vi "SubPanel_JSON_PowerConfiguration.vi"(3 "error_input":errorcluster, 4 "ColorPalette":T4=[16711686, 65351, 8978420, 14474240, 16139007, 16752640, 8958719, 16758973, 16777215, 46792, 11992992, 12961221, 16763690, 12600063, 16711835, 2953983, 40796, 13111296, 13352613, 9221011, 12964076, 12819897, 65442, 16776704, 14540253, 16740729, 10658047, 10813344, 16753521, 13413843, 8691115, 10339240, 14401205, 16746704, 7467519, 16775978, 13872558, 11387603, 13354405, 10420227, 13107364, 4060, 35208, 11817216, 7566080, 40796, 7539456, 2837073, 6372186, 7499083, 10648702, 16757152], 5 "VISAPowerInfoInputArray":T3[](array[typedef]), 6 "DCPowerInformationClusterArray_Input":T2[](array[typedef])) -> (0 "error output":errorcluster, 1 "VISAPowerInfoOutputArray":T3[](array[typedef]), 2 "DCPower_byInstrument_output":T1(array[cluster]))   [LabVIEW 2019]
uses:
  Controls/PlotColorArray.ctl
  Controls/VISA_power_Control.ctl
  Controls/DCPowerBlock_byInstrument_Control.ctl
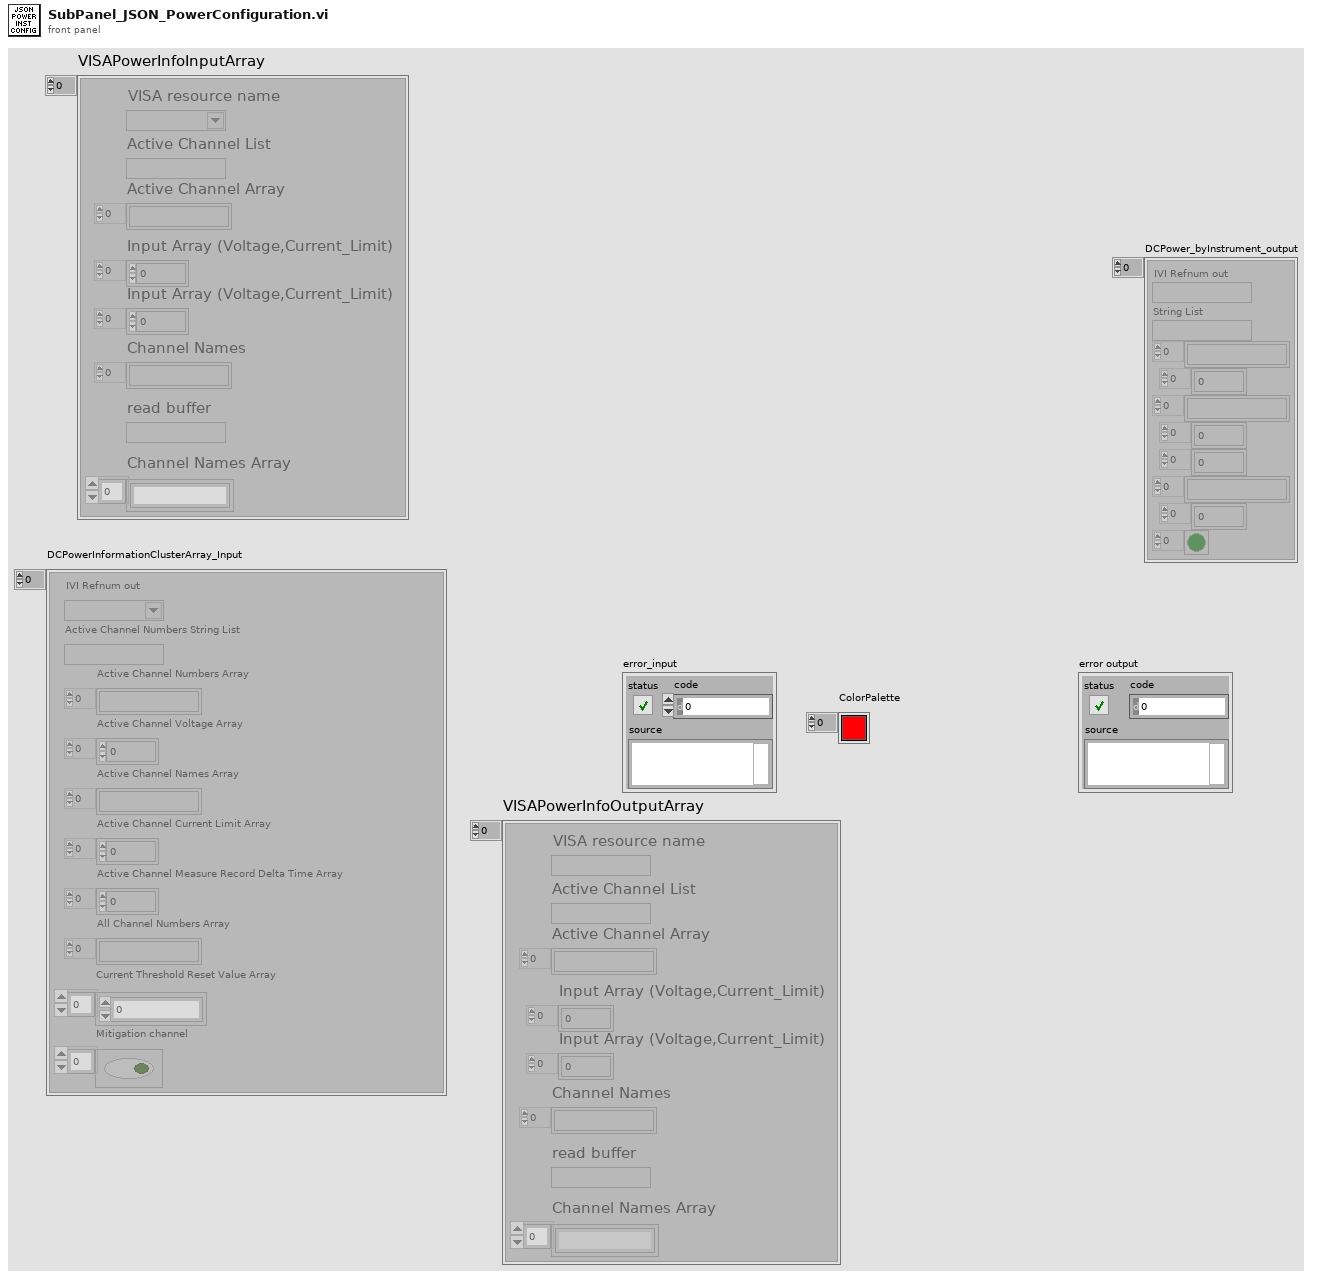
[diagram p1: front panel]
types:
  T1 = cluster{"IVI Refnum out":refnum<k15>, "String List":string, string[], dbl[], string[], dbl[], dbl[], string[], dbl[], bool[]}[]
  T2 = typedef "DCPowerBlock_byInstrument_Control.ctl" = cluster{"IVI Refnum out":refnum<k15>, "Active Channel Numbers String List":string, "Active Channel Numbers Array":string[], "Active Channel Voltage Array":dbl[], "Active Channel Names Array":string[], "Active Channel Current Limit Array":dbl[], "Active Channel Measure Record Delta Time Array":dbl[], "All Channel Numbers Array":string[], "Current Threshold Reset Value Array":dbl[], "Mitigation channel":bool[]}
  T3 = typedef "VISA_power_Control.ctl" = cluster{"VISA resource name":refnum<visa-resource-name>, "Active Channel List":string, "Active Channel Array":string[], "Input Array (Voltage,Current_Limit)":dbl[], "Input Array (Voltage,Current_Limit)":dbl[], "Channel Names":string[], "read buffer":string, "Channel Names Array":string[]}
  T4 = typedef "PlotColorArray.ctl" = u32[]
  T5 = cluster{"IVI Refnum out":refnum<k15>, "Active Channel Numbers String List":string, "Active Channel Numbers Array":string[], "Active Channel Voltage Array":dbl[], "Active Channel Names Array":string[], "Active Channel Current Limit Array":dbl[], "Active Channel Measure Record Delta Time Array":dbl[], "All Channel Numbers Array":string[], "Current Threshold Reset Value Array":dbl[], "Mitigation channel":bool[]}
  T6 = cluster{"IVI Refnum out":refnum<k15>, string, "voltage level channel 23":dbl, "Channel Name 23":string, "Current Limit":dbl, "Measure Record dt":dbl, string, "Current Threshold Reset Value Array":dbl, "Mitigation Channel":bool}[]
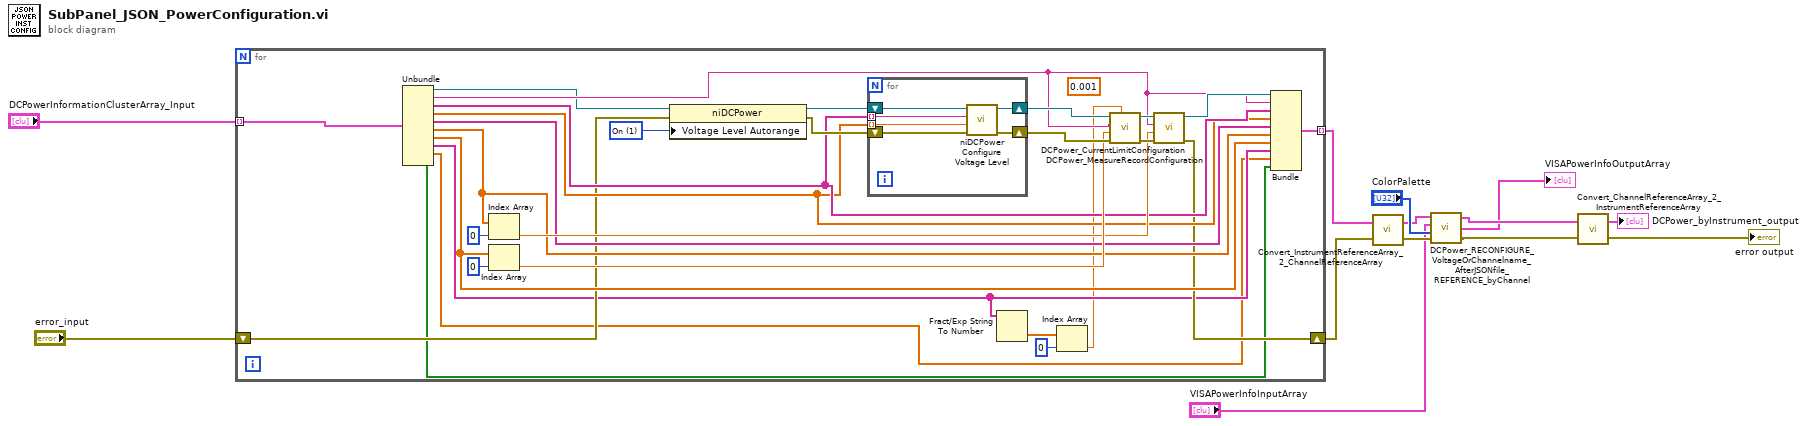
[diagram p0: block diagram]
diagram:
  n1 = for {
    tunnel: "DCPowerInformationClusterArray_Input" -> [w42] mode=indexing
    shift-right: [w20] -> w13
    shift-left: "error_input" -> [w21]
    tunnel: [w23] -> w12 mode=indexing
    (unwired) 0.001 ("Aperture Time")
    w41 = 1 items=["Off", "On"] ("Source:DC Voltage:Voltage Level Autorange")
    n2 = Unbundle(w42) -> ("IVI Refnum out"=w22:refnum<k15>, "Active Channel Numbers String List"=w29:string, "Active Channel Numbers Array"=w28:string[], "Active Channel Voltage Array"=w27:dbl[], "Active Channel Names Array"=w26:string[], "Active Channel Current Limit Array"=w25:dbl[], "Active Channel Measure Record Delta Time Array"=w24:dbl[], "All Channel Numbers Array"=w19:string[], "Current Threshold Reset Value Array"=w15:dbl[], "Mitigation channel"=w14:bool[])
    n3 = Index Array(array=w25, index=0) -> (element=w31:dbl)
    n4 = Index Array(array=w24, index=0) -> (element=w34:dbl)
    n5 = property class="niDCPower"(reference=w22, error in=w21, "Voltage Level Autorange"=w41) -> (reference out=w40:refnum<k15>, error out=w39:errorcluster)
    n6 = for {
      shift-right: [w48] -> w38
      shift-left: w39 -> [w46]
      shift-right: [w45] -> w37
      shift-left: w40 -> [w47]
      tunnel: w28 -> [w44] mode=indexing
      tunnel: w27 -> [w43] mode=indexing
      n7 = call <instrlib>:"niDCPower Configure Voltage Level.vi"("error in (no error)"=w46, "voltage level"=w43, "channel name"=w44, "instrument handle"=w47) -> ("error out"=w48:errorcluster, "instrument handle out"=w45:refnum<k15>)  [unwired: 6 in]
    }
    n8 = Fract/Exp String To Number(string=w19) -> (number=w17:dbl[])  [unwired: 3 in, 1 out]
    n9 = Index Array(array=w17, index=0) -> (element=w16:dbl)
    n10 = call "DCPower_MeasureRecordConfiguration.vi"("Aperture Time"=w16, "error in (no error)"=w38, "Measure Record Length"=w34, "Active Channel Numbers String"=w29, "IVI Refnum in"=w37) -> ("error out"=w33:errorcluster, "IVI Refnum out"=w32:refnum<k15>)  [unwired: 4 in, 1 out]
    n11 = call "DCPower_CurrentLimitConfiguration.vi"("error in (no error)"=w33, "current limit"=w31, "Active Channel Numbers String"=w29, "IVI Refnum in"=w32) -> ("error out"=w20:errorcluster, "IVI Refnum out"=w30:refnum<k15>)  [unwired: 6 in]
    n12 = Bundle("IVI Refnum out"=w30, "Active Channel Numbers String List"=w29, "Active Channel Numbers Array"=w28, "Active Channel Voltage Array"=w27, "Active Channel Names Array"=w26, "Active Channel Current Limit Array"=w25, "Active Channel Measure Record Delta Time Array"=w24, "All Channel Numbers Array"=w19, "Current Threshold Reset Value Array"=w15, "Mitigation channel"=w14) -> (w23:T5)  [unwired: 1 in]
  }
  n13 = call "Convert_InstrumentReferenceArray_2_ChannelReferenceArray.vi"("error in (no error)"=w13, "DCPowerInformationClusterArray_Input"=w12) -> ("error out"=w9:errorcluster, "DCPowerInformationArrayOutput_byChannel"=w2:T6)
  n14 = call "DCPower_RECONFIGURE_VoltageOrChannelname_AfterJSONfile_REFERENCE_byChannel.vi"("error in"=w9, "ColorPalette"="ColorPalette", "VISAPowerInfoInputArray"="VISAPowerInfoInputArray", "DCPowerInformationArrayOutput_byChannel_input"=w2) -> ("error out"=w6:errorcluster, "VISAPowerInfoOutputArray"=→"VISAPowerInfoOutputArray":T3[], "DCPowerInformationArrayOutput_byChannel_output"=w7:T6)
  n15 = call "Convert_ChannelReferenceArray_2_InstrumentReferenceArray.vi"("error in"=w6, "DCPowerInformation_byChannel_input"=w7) -> ("error out"=→"error output":errorcluster, "DCPower_byInstrument_output"=→"DCPower_byInstrument_output":T1)
